vi "Configure Resolution.vi"(8 "error in (no error)":errorcluster, 10 "Resolution":i32, 11 "RS Z2X in":refnum<class "RS Z2X.lvclass">) -> (0 "error out":errorcluster, 3 "RS Z2X out":refnum<class "RS Z2X.lvclass">)   [LabVIEW 2020, in "RS Z2X.lvclass"]
uses:
  RS Z2X.lvclass
  C:/Sandbox/RF Bench/Source Code/WiSpry Test Framework/Instruments/Instrument.lvclass
  Instrument.lvclass/Instrument.ctl
  Instrument.lvclass
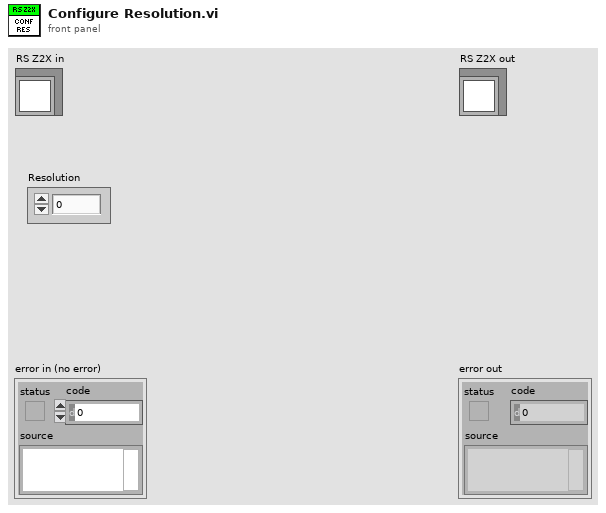
[diagram p1: front panel]
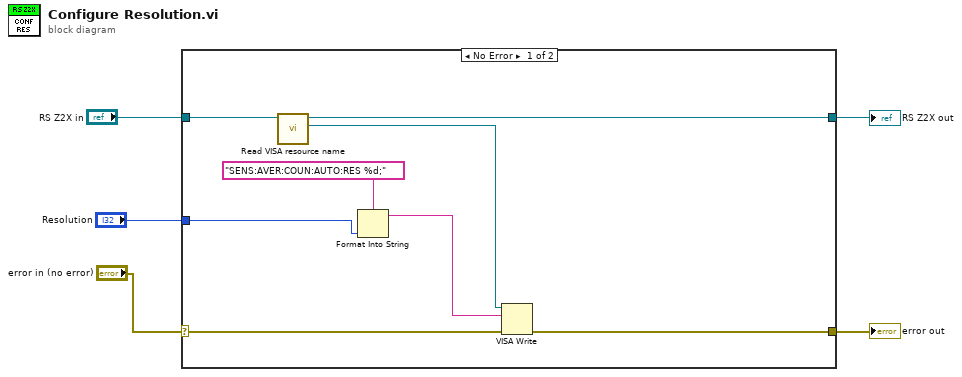
[diagram p0: block diagram]
diagram:
  n1 = case shown="No Error" "error in (no error)" {
    selector: "error in (no error)" -> [w9 w15]
    tunnel: [w8 w15] -> w4
    tunnel: [w12 w14] -> w3
    tunnel: "RS Z2X in" -> [w7 w14]
    tunnel: "Resolution" -> [w6 _]
    frame No Error {
      n2 = call "Read VISA resource name.vi"("Instrument in"=w7) -> ("VISA resource name"=w13:refnum<visa-resource-name>, "Instrument out"=w12:refnum<class "RS Z2X.lvclass">)  [unwired: 9 in]
      n3 = Format Into String(format string="SENS:AVER:COUN:AUTO:RES %d;", w6) -> (resulting string=w10:string)  [unwired: 2 in, 1 out]
      n4 = VISA Write(VISA resource name=w13, write buffer=w10, error in (no error)=w9) -> (error out=w8:errorcluster)  [unwired: 2 out]
    }
    frame Error {
    }
  }
  "error out" <- w4
  "RS Z2X out" <- w3
